vi "test.vi"() -> ()   [LabVIEW 2020]
panel:
  in  "cb test":bool
  in  "objd":string
  in  "objc":string
  in  "btn exit":bool
  in  "objb":string
  in  "obja":string
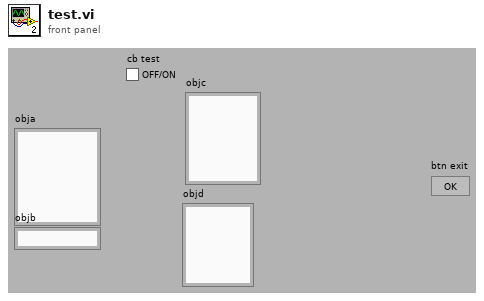
[diagram p1: front panel]
types:
  T1 = typedef "LVRectTypeDef.ctl" = cluster{"Left":i16, "Top":i16, "Right":i16, "Bottom":i16}
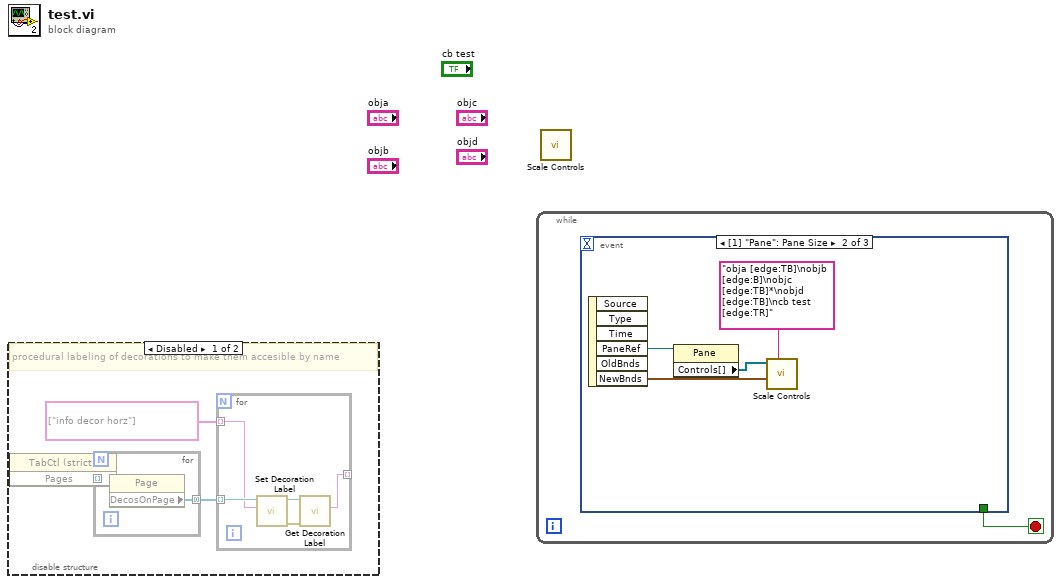
[diagram p0: block diagram]
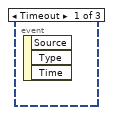
[diagram p3: hidden frame]
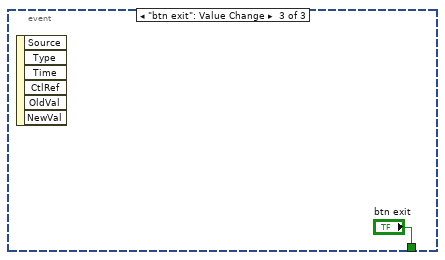
[diagram p4: hidden frame]
diagram:
  n1 = disable-structure shown="Disabled" {
    frame Disabled {
      # "procedural labeling of decorations to make them accesible by name"
      n2 = property on="Property Node" class="TabCtl (strict)"() -> ("Pages"=w3:refnum<vi>[])  [unwired: 2 in, 2 out]
      n3 = for {
        tunnel: w3 -> [w10] mode=indexing
        tunnel: [w9] -> w2 mode=concatenating
        n4 = property class="Page"(reference=w10) -> ("DecosOnPage"=w9:refnum<vi>[])  [unwired: 1 in, 2 out]
      }
      n5 = for {
        tunnel: w2 -> [w8] mode=indexing
        tunnel: string[] ["info decor horz"] -> [w7] mode=indexing
        tunnel: [w4] -> _ mode=indexing
        n6 = call "Set Decoration Label.vi"("Label"=w7, "Decor Refnum"=w8) -> ("error out"=w6:errorcluster, "dup Decor Refnum"=w5:refnum<vi>)  [unwired: 4 in]
        n7 = call "Get Decoration Label.vi"("error in"=w6, "Decor Refnum"=w5) -> ("Label"=w4:string)  [unwired: 3 in, 2 out]
      }
    }
    frame Enabled {
    }
  }
  n8 = while {
    stop <- w11 stop-if-true
    n9 = event shown="[1] \"Pane\": Pane Size" {
      selector: _ -> [_ _ _]
      dyn-events: _ -> [_ _ _]
      timeout: _ -> [_ _ _]
      tunnel: [_ _ "btn exit"] -> w11
      event Timeout {
        n10 = event-data() -> ()  [unwired: 1 in, 3 out]
      }
      event Pane Size {
        n11 = event-data() -> ("PaneRef"=w14:refnum<vi>, "NewBnds"=w15:T1)  [unwired: 1 in, 4 out]
        n12 = property class="Pane"(reference=w14) -> ("Controls[]"=w13:refnum<vi>[])  [unwired: 1 in, 2 out]
        n13 = call "Scale Controls.vi"("rules"="obja [edge:TB]\nobjb [edge:B]\nobjc [edge:TB]*\nobjd [edge:TB]\ncb test [edge:TR]", "pane size"=w15, "Controls on Pane"=w13) -> ()  [unwired: 8 in, 1 out]
      }
      event "btn exit": Value Change {
        n14 = event-data() -> ()  [unwired: 1 in, 6 out]
      }
    }
  }
  n15 = call "Scale Controls.vi"() -> ()  [unwired: 11 in, 1 out]
